vi "CTE_Analysis_Suite_InputMaker_FormatHKL.vi"(11 "HKLs and D-Spacings":string) -> (3 "Output":string)   [LabVIEW 2012]
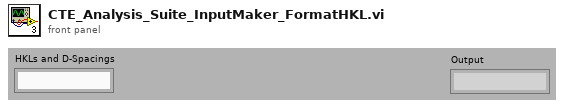
[diagram p1: front panel]
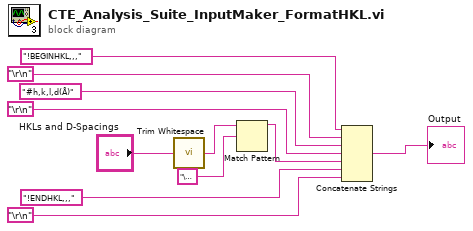
[diagram p0: block diagram]
diagram:
  n1 = call <vilib>:"Trim Whitespace.vi"("string"="HKLs and D-Spacings") -> ("trimmed string"=w1:string)  [unwired: 1 in]
  n2 = Match Pattern(string=w1, regular expression="\u0000" ("string")) -> (before substring=w3:string)  [unwired: 1 in, 3 out]
  n3 = Concatenate Strings("!BEGINHKL,,,", "\r\n", "#h,k,l,d(Å)", "\r\n", w3, "!ENDHKL,,,", "\r\n") -> (→"Output":string)
